vi "for_loop_timer.vi"() -> ()   [LabVIEW 2025]
panel:
  out "d0":bool
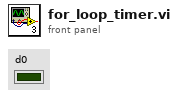
[diagram p1: front panel]
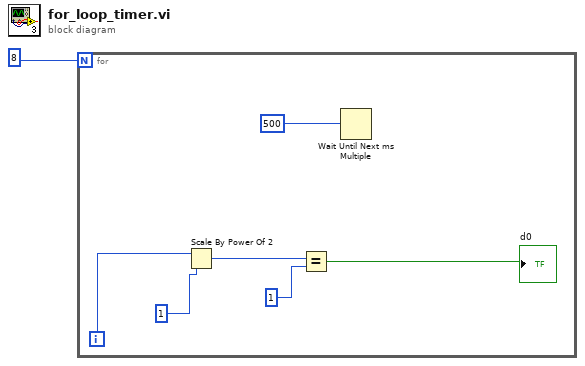
[diagram p0: block diagram]
diagram:
  n1 = for {
    N: 8 -> [_]
    i -> [w3]
    n2 = Scale By Power Of 2(n=w3, x=1) -> (x*2^n=w2:i32)
    n3 = Equal?(x=w2, y=1) -> (x = y?=→"d0":bool)
    n4 = Wait Until Next ms Multiple(millisecond multiple=500) -> ()  [unwired: 1 out]
  }
